vi "Read Write LS App Config.vi"(7 "Write (F)":bool, 8 "Error IN":errorcluster, 10 "LS App Config In":T1={"LS Power (Freq):"=0.0, "LS Power (Duty):"=0.0, "Bank 1 Present"={"1"=TRUE, "2"=TRUE, "3"=TRUE, "4"=TRUE, "5"=TRUE}, "Bank 2 Present"={"6"=TRUE, "7"=TRUE, "8"=TRUE, "9"=TRUE, "10"=TRUE}, "Data File Name:"="", "Record Bursts"=FALSE, "RecInterval(s)"=600, "RecDuration(s)"=10, "RecFrequeny (Hz)"=1000, "DetectionMode"=0, "Serial Numbers"=["", "", "", "", "", "", "", "", "", "", "", ""], "Record Constant"=FALSE, "2nd Step Check"=FALSE, "Bias Resistances"=[681.0, 681.0, 681.0, 681.0, 681.0, 681.0, 681.0, 681.0, 681.0, 681.0, 681.0, 681.0], "Voltage(T)/Resistance(F)"=TRUE}, 11 "Refnum in":T2) -> (0 "Error OUT":errorcluster, 2 "LS App Config Out":T1={"LS Power (Freq):"=0.0, "LS Power (Duty):"=0.0, "Bank 1 Present"={"1"=TRUE, "2"=TRUE, "3"=TRUE, "4"=TRUE, "5"=TRUE}, "Bank 2 Present"={"6"=TRUE, "7"=TRUE, "8"=TRUE, "9"=TRUE, "10"=TRUE}, "Data File Name:"="", "Record Bursts"=FALSE, "RecInterval(s)"=600, "RecDuration(s)"=10, "RecFrequeny (Hz)"=1000, "DetectionMode"=0, "Serial Numbers"=["", "", "", "", "", "", "", "", "", "", "", ""], "Record Constant"=FALSE, "2nd Step Check"=FALSE, "Bias Resistances"=[681.0, 681.0, 681.0, 681.0, 681.0, 681.0, 681.0, 681.0, 681.0, 681.0, 681.0, 681.0], "Voltage(T)/Resistance(F)"=TRUE}, 3 "Refnum out":T2)   [LabVIEW 2013]
uses:
  <vilib>/Utility/config.llb/Config Data RefNum.ctl
  <vilib>/Utility/config.llb/NI_LVConfig.lvlib
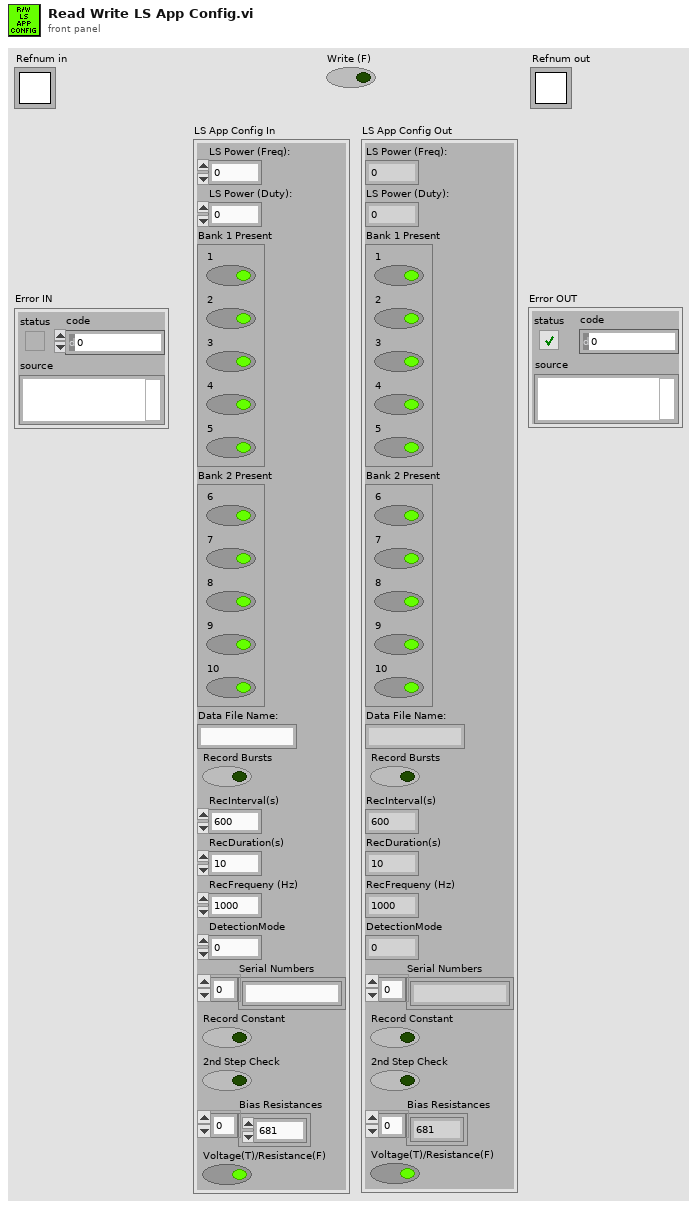
[diagram p1: front panel]
types:
  T1 = cluster{"LS Power (Freq):":dbl, "LS Power (Duty):":dbl, "Bank 1 Present":cluster{"1":bool, "2":bool, "3":bool, "4":bool, "5":bool}, "Bank 2 Present":cluster{"6":bool, "7":bool, "8":bool, "9":bool, "10":bool}, "Data File Name:":string, "Record Bursts":bool, "RecInterval(s)":i32, "RecDuration(s)":i32, "RecFrequeny (Hz)":i32, "DetectionMode":i32, "Serial Numbers":string[], "Record Constant":bool, "2nd Step Check":bool, "Bias Resistances":dbl[], "Voltage(T)/Resistance(F)":bool}
  T2 = typedef "NI_LVConfig.lvlib/Config Data RefNum.ctl" = refnum<k1>
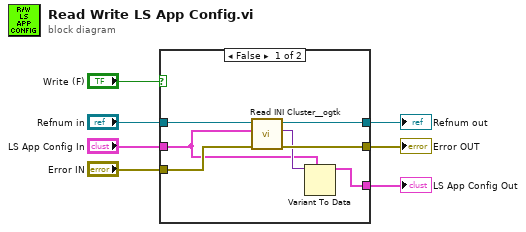
[diagram p0: block diagram]
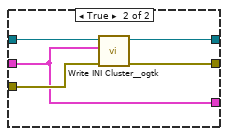
[diagram p2: hidden frame]
diagram:
  n1 = case shown="False" "Write (F)" {
    tunnel: "Refnum in" -> [w14 w19]
    tunnel: "LS App Config In" -> [w10 w16]
    tunnel: "Error IN" -> [w13 w18]
    tunnel: [w8 w17] -> w4
    tunnel: [w9 w16] -> w1
    tunnel: [w12 w15] -> w5
    frame False {
      n2 = call <userlib>:"Read INI Cluster__ogtk.vi"("error in (no error)"=w13, "INI Fomatted Cluster Type"=w10, "refnum"=w14) -> ("error out"=w12:errorcluster, "INI Fomatted Cluster"=w11:variant, "dup refnum"=w8:T2)  [unwired: 4 in, 2 out]
      n3 = Variant To Data(type=w10, Variant=w11) -> (data=w9:T1)  [unwired: 1 in, 1 out]
    }
    frame True {
      n4 = call <userlib>:"Write INI Cluster__ogtk.vi"("error in (no error)"=w18, "INI Fomatted Cluster"=w16, "refnum"=w19) -> ("error out"=w15:errorcluster, "dup refnum"=w17:T2)  [unwired: 7 in]
    }
  }
  "Error OUT" <- w5
  "Refnum out" <- w4
  "LS App Config Out" <- w1
